vi "Vehicle out of Position Update.vi"(8 "error in (no error)":errorcluster, 10 "Vehicle ouf ot Position":bool, 11 "Fancy Car Position Simulation View in":refnum<class "Fancy Car Position Simulation View.lvclass">) -> (0 "error out":errorcluster, 3 "Fancy Car Position Simulation View out":refnum<class "Fancy Car Position Simulation View.lvclass">)   [LabVIEW 2019, in "Fancy Car Position Simulation View.lvclass"]
uses:
  <vilib>/gpm_packages/@cs/Car-wash/Source/Fancy Car Position Simulation View/Fancy Car Position Simulation View/Fancy Car Position Simulation View.lvclass
  C:/Program Files/National Instruments/LabVIEW 2019/vi.lib/gpm_packages/@cs/Car-wash/Source/Car Position Simulation View Definition/Car Position Simulation View Definition/Car Position Simulation View Definition.lvclass
  <vilib>/gpm_packages/@cs/Car-wash/Source/Car Position Simulation View Definition/Car Position Simulation View Definition/Car Position Simulation View Definition.lvclass/Car Position Simulation View Definition.ctl
  <vilib>/gpm_packages/@cs/Car-wash/Source/Car Position Simulation View Definition/Car Position Simulation View Definition/Car Position Simulation View Definition.lvclass
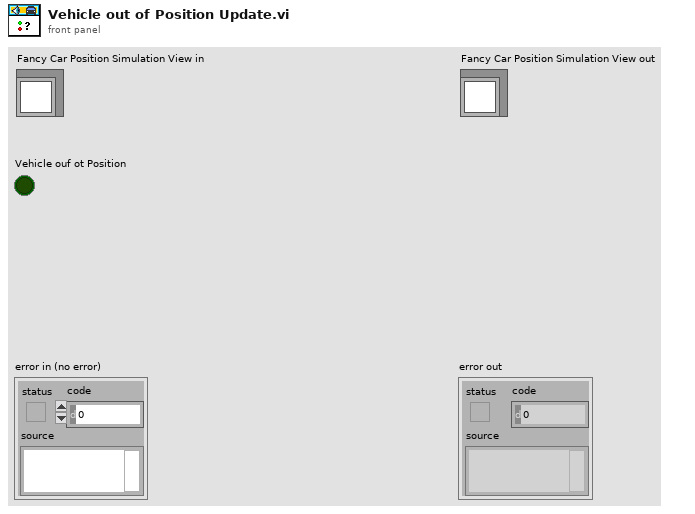
[diagram p1: front panel]
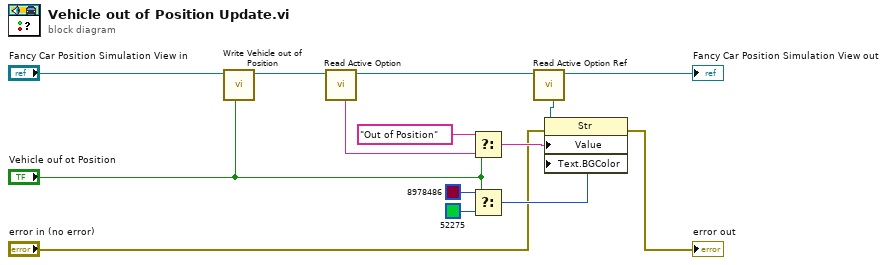
[diagram p0: block diagram]
diagram:
  n1 = call <vilib>:"Write Vehicle out of Position.vi"("Vehicle out of Position"="Vehicle ouf ot Position", "Car Position Simulation View Definition in"="Fancy Car Position Simulation View in") -> ("Car Position Simulation View Definition out"=w2:refnum<class "Fancy Car Position Simulation View.lvclass">)  [unwired: 9 in]
  n2 = call <vilib>:"Read Active Option.vi"("Car Position Simulation View Definition in"=w2) -> ("Car Position Simulation View Definition out"=w13:refnum<class "Fancy Car Position Simulation View.lvclass">, "Active Option"=w11:string)  [unwired: 9 in]
  n3 = Select(t="Out of Position", s="Vehicle ouf ot Position", f=w11) -> (s? t:f=w9:string)
  n4 = Select(t=u32 8978486, s="Vehicle ouf ot Position", f=u32 52275) -> (s? t:f=w6:u32)
  n5 = call <vilib>:"Read Active Option Ref.vi"("Car Position Simulation View Definition in"=w13) -> ("Car Position Simulation View Definition out"=→"Fancy Car Position Simulation View out":refnum<class "Fancy Car Position Simulation View.lvclass">, "Active Option Ref"=w12:refnum<vi>)  [unwired: 9 in]
  n6 = property class="Str"(reference=w12, error in="error in (no error)", "Value"=w9, "Text.BGColor"=w6) -> (error out=→"error out":errorcluster)  [unwired: 1 out]
